vi "PostBookingInstrument.vi"(8 "error in (no error)":errorcluster, 10 "BookingInstrument":T1, 11 "ByteGSWebAPI-V0 in":refnum<class "ByteGSWebAPI-V0.lvclass">) -> (0 "error out":errorcluster, 3 "ByteGSWebAPI-V0 out":refnum<class "ByteGSWebAPI-V0.lvclass">)   [LabVIEW 2019, in "ByteGSWebAPI-V0.lvclass"]
uses:
  ByteGSWebAPI-V0.lvclass
  1f9a4a84-1e23-43aa-b54f-cc03f7d81dac.vi
  Cntrls/PostBooking.ctl
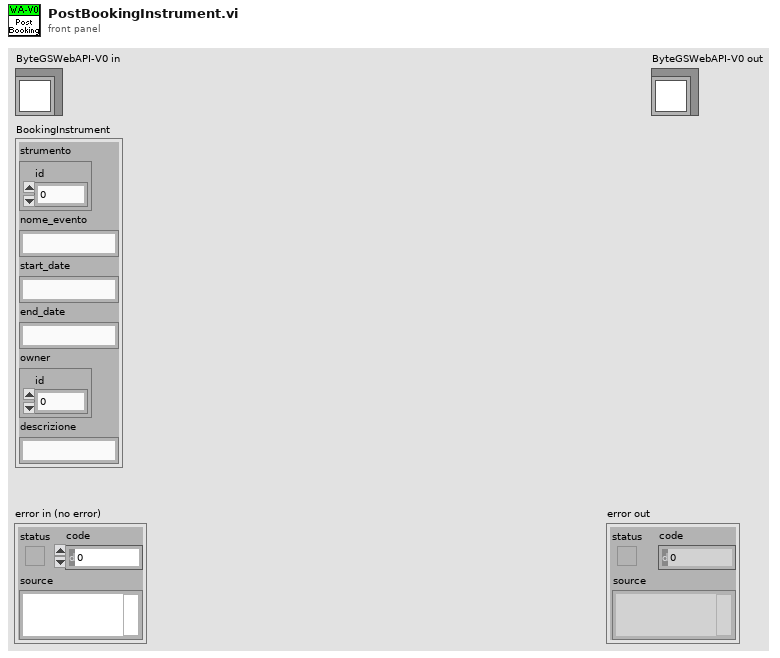
[diagram p1: front panel]
types:
  T1 = typedef "ByteGSWebAPI-V0.lvclass/PostBooking.ctl" = cluster{"strumento":cluster{"id":i32}, "nome_evento":string, "start_date":string, "end_date":string, "owner":cluster{"id":i32}, "descrizione":string}
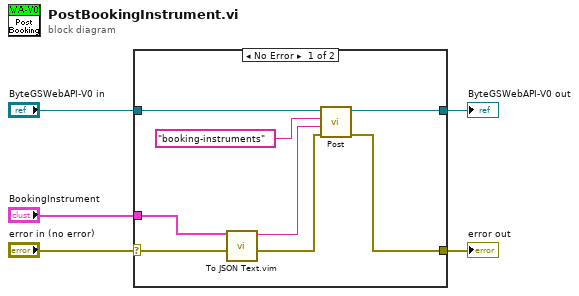
[diagram p0: block diagram]
diagram:
  n1 = case shown="No Error" "error in (no error)" {
    selector: "error in (no error)" -> [w11 w15]
    tunnel: [w7 w15] -> w4
    tunnel: [w13 w14] -> w2
    tunnel: "ByteGSWebAPI-V0 in" -> [w12 w14]
    tunnel: "BookingInstrument" -> [w6 _]
    frame No Error {
      n2 = call "To JSON Text.vim"("error in (no error)"=w11, "Anything"=w6) -> ("error out"=w10:errorcluster, "<JSON>"=w9:string)  [unwired: 8 in]
      n3 = call "Post.vi"("error in (no error)"=w10, "Buffer"=w9, "Request"="booking-instruments", "ByteGSWebAPI-V0 in"=w12) -> ("error out"=w7:errorcluster, "ByteGSWebAPI-V0 out"=w13:refnum<class "ByteGSWebAPI-V0.lvclass">)  [unwired: 4 in, 2 out]
    }
    frame Error {
    }
  }
  "error out" <- w4
  "ByteGSWebAPI-V0 out" <- w2
